vi "Update Chnls Sync.vi"(8 "error in (no error)":errorcluster, 10 "ChnlSettings":T1[](array[typedef]) {"ChnParameter"."Delay (µs)" min=0.0 max=100000000.0 format="%.4f"; "G08_Chnl_Settings"."Pulse Width (µs)" min=0.0 max=8947840.0 format="%#.6f"; "Go and Done Signal"."Done Signal" format="%04x" items=["Local Primary"=1, "Local Secondary"=2, "Local Force"=4, "Master Primary"=16]; "Go and Done Signal"."Go Signal" format="%04x" items=["Local Primary0x1"=1, "Local Secondary0x2"=2, "Local Force 0x4"=4, "Resynchronize 0x8"=8, "Master Prim. 0x10"=16, "Master Sec. 0x20"=32, "Master Force  0x40"=64, "System Clock 0x80"=128, "Delay Clock 0x100"=256, "Inhibit Local 0x200"=512, "Start Local 0x400"=1024, "Start Bus 0x800"=2048, "Step Back Local 0x1000"=4096, "Step Back Bus 0x2000"=8192, "RunCircle 0x4000"=16384, "SyncReload 0x8000"=32768, "From E 0x10000"=65536, "From F 0x20000"=131072, "From Bus 0x40000"=262144]}, 11 "BME_DG_System in":refnum<class "BME_DG_System.lvclass">) -> (0 "error out":errorcluster, 2 "ProblemChnls":string[](array[string]), 3 "BME_DG_System out":refnum<class "BME_DG_System.lvclass">)   [LabVIEW 2009, in "POLARIS BME DG.lvlib" / "BME_DG_System.lvclass"]
uses:
  BME_DG_System.lvclass
  Chnl Settings Complete.ctl
  LV-BME Interface/ChnlSettings.ctl
  Go_Done_Chnl_Settings.ctl
  MSBus.ctl
  SG08_Chnl_Settings.ctl
  BME_DG_Chnl/BME_DG_Chnl.lvclass
  POLARIS BME DG.lvlib
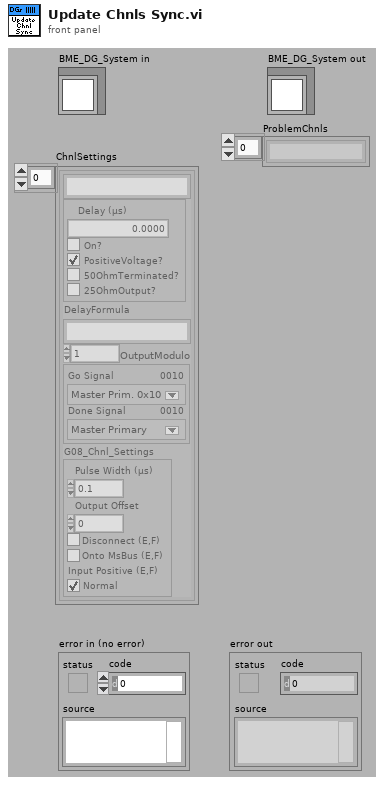
[diagram p1: front panel]
types:
  T1 = typedef "POLARIS BME DG.lvlib/Chnl Settings Complete.ctl" = cluster{"Channel Name":string, "ChnParameter":T2, "DelayFormula":string, "OutputModulo":i32, "Go and Done Signal":T3, "G08_Chnl_Settings":T5}
  T2 = typedef "POLARIS BME DG.lvlib/ChnlSettings.ctl" = cluster{" Delay (µs)":dbl, "On?":bool, "PositiveVoltage?":bool, "50OhmTerminated? ":bool, "25OhmOutput?":bool}
  T3 = typedef "POLARIS BME DG.lvlib/Go_Done_Chnl_Settings.ctl" = cluster{"Go Signal":T4, "Done Signal":u32}
  T4 = typedef "POLARIS BME DG.lvlib/MSBus.ctl" = u32
  T5 = typedef "POLARIS BME DG.lvlib/SG08_Chnl_Settings.ctl" = cluster{"Pulse Width (µs)":dbl, "Output Offset":u32, "Disconnect (E,F)":bool, "Onto MsBus (E,F)":bool, "Input Positive (E,F)":bool}
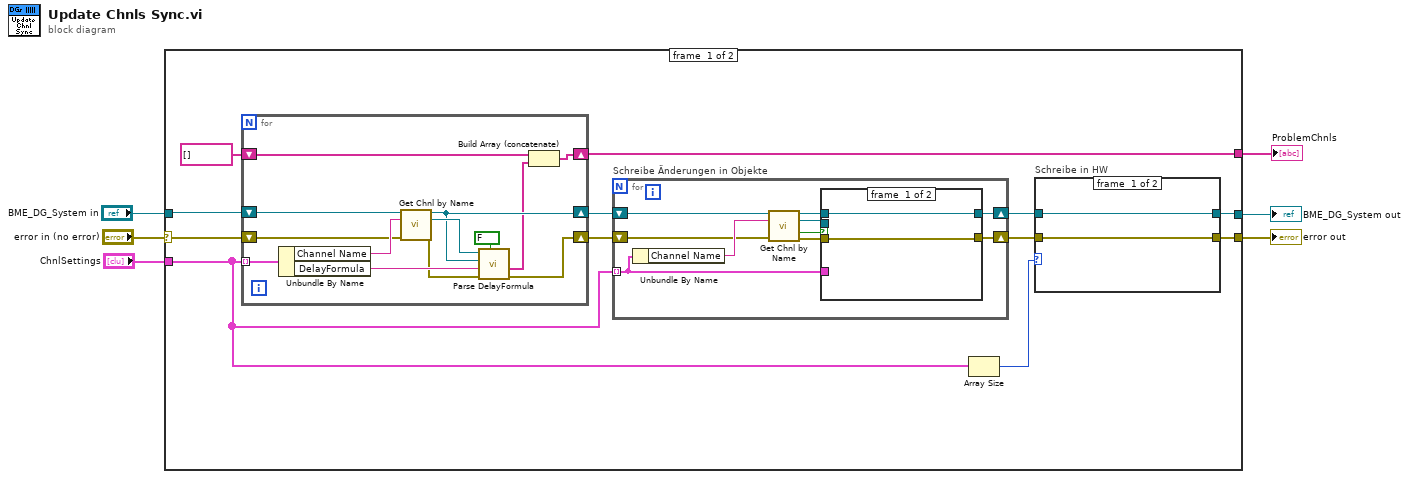
[diagram p0: block diagram]
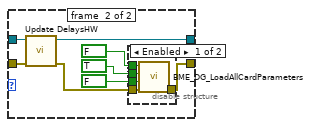
[diagram p2: hidden frame]
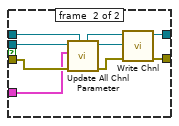
[diagram p4: hidden frame]
diagram:
  n1 = case shown="No Error" "error in (no error)" {
    selector: "error in (no error)" -> [w12 w70]
    tunnel: [w8 w70] -> w6
    tunnel: [w9 w69] -> w5
    tunnel: "BME_DG_System in" -> [w15 w69]
    tunnel: "ChnlSettings" -> [w13 _]
    tunnel: [w10 _] -> w1
    frame #0 {
      n2 = for {
        tunnel: w13 -> [w24] mode=indexing
        shift-right: [w25] -> w14
        shift-left: w15 -> [w26]
        shift-right: [w22] -> w11
        shift-left: w12 -> [w23]
        shift-right: [w20] -> w10
        shift-left: string[] [] -> [w19]
        n3 = Unbundle By Name(w24) -> ("Channel Name"=w27:string, "DelayFormula"=w30:string)
        n4 = call "Get Chnl by Name.vi"("BME_DG_System in"=w26, "Chnl Name"=w27, "error in (no error)"=w23) -> ("BME_DG_System out"=w25:refnum<class "BME_DG_System.lvclass">, "BME_DG_Chnl"=w28:refnum<class "BME_DG_Chnl.lvclass">, "error out"=w29:errorcluster)  [unwired: 7 in, 3 out]
        n5 = call "Parse DelayFormula.vi"("UpdateChnlObjects?"=FALSE, "error in (no error)"=w29, "DelayFormula"=w30, "BME_DG_System"=w25, "BME_DG_Chnl in"=w28) -> ("error out"=w22:errorcluster, "Problem Chnls out"=w21:string[])  [unwired: 3 in, 2 out]
        n6 = Build Array (concatenate)(w19, w21) -> (w20:string[])
      }
      n7 = for "Schreibe Änderungen in Objekte" {
        shift-right: [w52] -> w17
        shift-left: w14 -> [w53]
        tunnel: w13 -> [w48] mode=indexing
        shift-right: [w49] -> w16
        shift-left: w11 -> [w50]
        n8 = Unbundle By Name(w48) -> ("Channel Name"=w51:string)
        n9 = call "Get Chnl by Name.vi"("BME_DG_System in"=w53, "Chnl Name"=w51, "error in (no error)"=w50) -> ("BME_DG_System out"=w55:refnum<class "BME_DG_System.lvclass">, "BME_DG_Chnl"=w56:refnum<class "BME_DG_Chnl.lvclass">, "found?"=w57:bool, "error out"=w54:errorcluster)  [unwired: 7 in, 2 out]
        n10 = case shown="True" w57 {
          tunnel: w56 -> [_ w65]
          tunnel: w55 -> [w59 w63]
          tunnel: w54 -> [w58 w66]
          tunnel: [w59 w67] -> w52
          tunnel: [w58 w68] -> w49
          tunnel: w48 -> [_ w64]
          frame #0 {
          }
          frame #1 {
            n11 = call "Update All Chnl Parameter.vi"("BME_DG_System in"=w63, "error in (no error)"=w66, "ChnlSettings"=w64, "BME_DG_Chnl in"=w65) -> ("error out"=w61:errorcluster, "BME_DG_Chnl out"=w60:refnum<class "BME_DG_Chnl.lvclass">, "BME_DG_System out"=w62:refnum<class "BME_DG_System.lvclass">)  [unwired: 5 in]
            n12 = call "Write Chnl.vi"("error in (no error)"=w61, "BME_DG_Chnl.lvclass"=w60, "BME_DG_System in"=w62) -> ("error out"=w68:errorcluster, "BME_DG_System out"=w67:refnum<class "BME_DG_System.lvclass">)  [unwired: 7 in]
          }
        }
      }
      n13 = Array Size(array=w13) -> (size(s)=w18:i32)
      n14 = case "Schreibe in HW" shown="1, Default" w18 {
        tunnel: [w33 w37] -> w9
        tunnel: [w32 w38] -> w8
        tunnel: w17 -> [w33 w41]
        tunnel: w16 -> [w32 w40]
        frame #0 {
        }
        frame #1 {
          n15 = call "Update DelaysHW.vi"("error in (no error)"=w40, "BME_DG_System in"=w41) -> ("error out"=w39:errorcluster, "BME_DG_System out"=w37:refnum<class "BME_DG_System.lvclass">)  [unwired: 8 in]
          n16 = disable-structure shown="Enabled" {
            disable-tunnel: w39 -> [w46 w47]
            disable-tunnel: [w45 w47] -> w38
            disable-tunnel: FALSE ("TimeList") -> [w44 _]
            disable-tunnel: TRUE ("ModuloCounter") -> [w43 _]
            disable-tunnel: FALSE ("EventCounter") -> [w42 _]
            frame #0 {
              n17 = call "BME_DG_LoadAllCardParameters.vi"("error in (no error)"=w46, "TimeList"=w44, "ModuloCounter"=w43, "EventCounter"=w42) -> ("error out"=w45:errorcluster)  [unwired: 7 in]
            }
            frame #1 {
            }
          }
        }
      }
    }
    frame #1 {
    }
  }
  "error out" <- w6
  "BME_DG_System out" <- w5
  "ProblemChnls" <- w1
